vi "Player Info.vi"(11 "Line Dancer in":refnum<class "Bricks.lvclass">) -> (1 "Victory Speech":string, 2 "Name":string, 3 "Line Dancer out":refnum<class "Bricks.lvclass">)   [LabVIEW 2015, in "Bricks.lvclass"]
uses:
  Bricks.lvclass
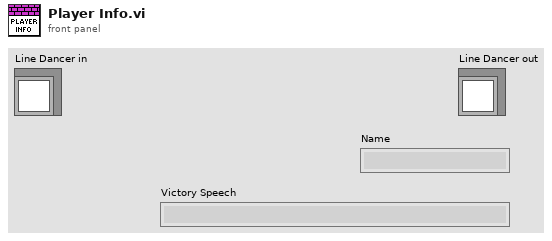
[diagram p1: front panel]
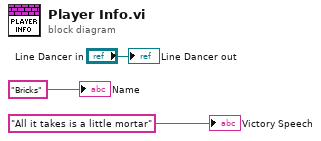
[diagram p0: block diagram]
diagram:
  "Line Dancer out" <- "Line Dancer in"
  "Name" <- "Bricks" ("Name")
  "Victory Speech" <- "All it takes is a little mortar" ("Victory Speech")
